vi "Init.vi"(10 "State":refnum<vi>) -> (3 "Constellation Command Handler out":refnum<class "Constellation Command Handler.lvclass">)   [LabVIEW 2023, in "VectoScratch.lvlib" / "Constellation Command Handler.lvclass"]
uses:
  Constellation Command Handler.lvclass
  Constellation Command Handler.lvclass/Constellation Command Handler.ctl
  Vecto/proto/ConstellationCommand/Data.ctl
  Vecto/proto/ConstellationCommand/ConstellationCommand.lvlib
  Vecto/Connection State.ctl
  Vecto/Vecto.lvlib
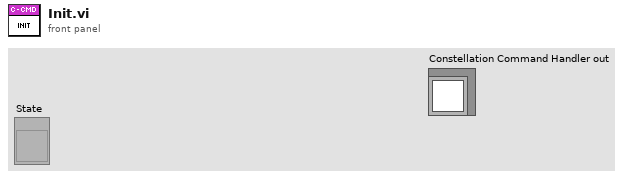
[diagram p1: front panel]
types:
  T1 = typedef "ConstellationCommand.lvlib/Data.ctl" = cluster{"Target Module":string, "Command":string, "Data":string[], "Time Stamp":timestamp}
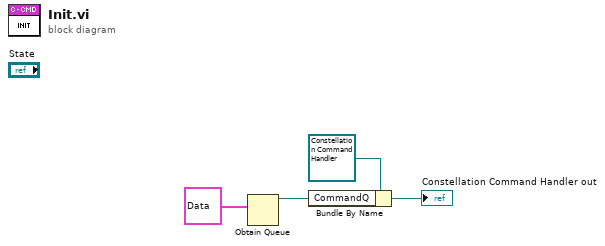
[diagram p0: block diagram]
diagram:
  n1 = Obtain Queue(element data type=T1 {"Target Module"="", "Command"="", "Data"=[], "Time Stamp"=timestamp(0 s since 1904-01-01)} ("Command Data")) -> (queue out=w1:refnum<queue>)  [unwired: 4 in, 2 out]
  n2 = Bundle By Name(cluster=refnum<class "Constellation Command Handler.lvclass"> refnum ("VectoScratch.lvlib:Constellation Command Handler.lvclass"), "CommandQ"=w1) -> (→"Constellation Command Handler out":refnum<class "Constellation Command Handler.lvclass">)
